vi "Toggle Example.vi"() -> ()   [LabVIEW 2012]
uses:
  <vilib>/Rock Robotics/WPI/Joystick/WPI_JoystickGetSetRefNum.vi
panel:
  out "Boolean":bool
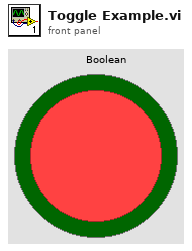
[diagram p1: front panel]
types:
  T1 = typedef "WPI_JoystickDevRef.ctl" = cluster{"Device":T2}
  T2 = typedef "WPI_JoystickDeviceEnum.ctl" = enum16{"USB 1", "USB 2", "USB 3", "USB 4", "Kinect 1", "Kinect 2"}
  T3 = typedef "WPI_JoystickButtonState.ctl" = cluster{"Button 1":bool, "Button 2":bool, "Button 3":bool, "Button 4":bool, "Button 5":bool, "Button 6":bool, "Button 7":bool, "Button 8":bool, "Button 9":bool, "Button 10":bool, "Button 11":bool, "Button 12":bool}
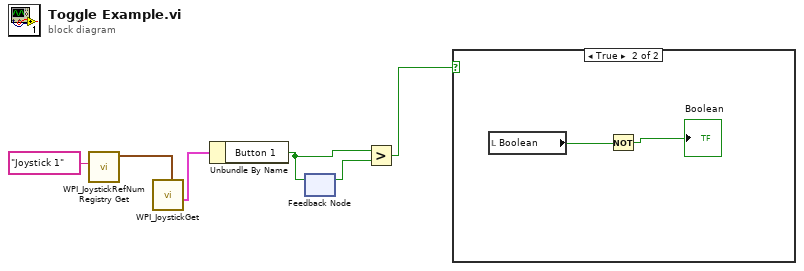
[diagram p0: block diagram]
diagram:
  n1 = call <vilib>:"WPI_JoystickRefNum Registry Get.vi"("refnum name"="Joystick 1") -> ("JoystickDevRef"=w5:T1)  [unwired: 9 in, 1 out]
  n2 = call <vilib>:"WPI_JoystickGet.vi"("JoystickDevRef"=w5) -> ("Buttons"=w4:T3)  [unwired: 4 in, 2 out]
  n3 = Unbundle By Name(w4) -> ("Button 1"=w2:bool)
  n4 = feedback-in #1(w2) -> ()
  n5 = feedback #1() -> (w3:bool)  [unwired: 1 in]
  n6 = Greater?(x=w2, y=w3) -> (0:w6:bool)
  n7 = case shown="True" w6 {
    frame False {
    }
    frame True {
      n8 = local read "Boolean"() -> (w7:bool)
      n9 = Not(x=w7) -> (.not. x?=→"Boolean":bool)
    }
  }
